vi "setPropertyIntValue.vi"(8 "error in (no error)":errorcluster, 9 "Property Value in":i32, 10 "Property Name in":string, 11 "IPropertyObject in":refnum<class "IPropertyObject.lvclass">) -> (0 "error out":errorcluster, 1 "Property Value out":i32, 2 "Property Name out":string, 3 "IPropertyObject out":refnum<class "IPropertyObject.lvclass">)   [LabVIEW 2022 SP3, in "openDAQ.lvlib" / "IBaseObject.lvlib" / "IPropertyObject.lvlib" / "IPropertyObject.lvclass"]
uses:
  <instrlib>/openDAQ/Public/Classes/IPropertyObject/IPropertyObject.lvclass
  C:/Program Files (x86)/National Instruments/LabVIEW 2022/instr.lib/openDAQ/Public/Classes/IBaseObject/IBaseObject.lvclass
  <instrlib>/openDAQ/Public/Classes/IBaseObject/IBaseObject.lvclass/IBaseObject.ctl
  <instrlib>/openDAQ/Public/Classes/IBaseObject/Accessor/Read reference.vi
  <instrlib>/openDAQ/Public/Classes/IBaseObject/Accessor/Write reference.vi
  <instrlib>/openDAQ/Public/Classes/daqCoreTypes/IInteger/IInteger.lvclass
  <instrlib>/openDAQ/Public/Classes/daqCoreTypes/IString/IString.lvclass
  <instrlib>/openDAQ/Binaries/Windows/x86/copendaq32.dll
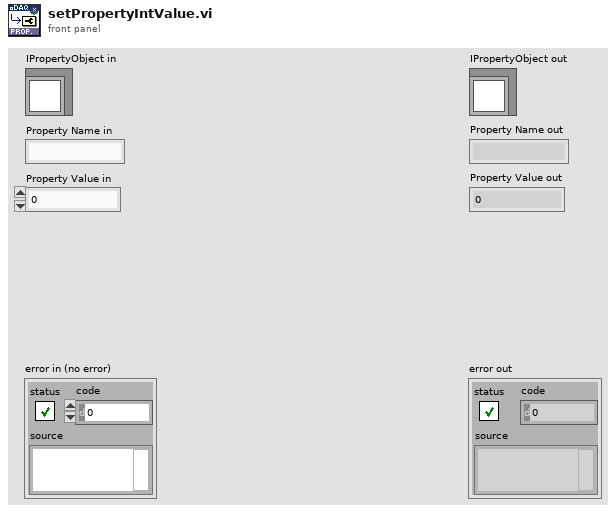
[diagram p1: front panel]
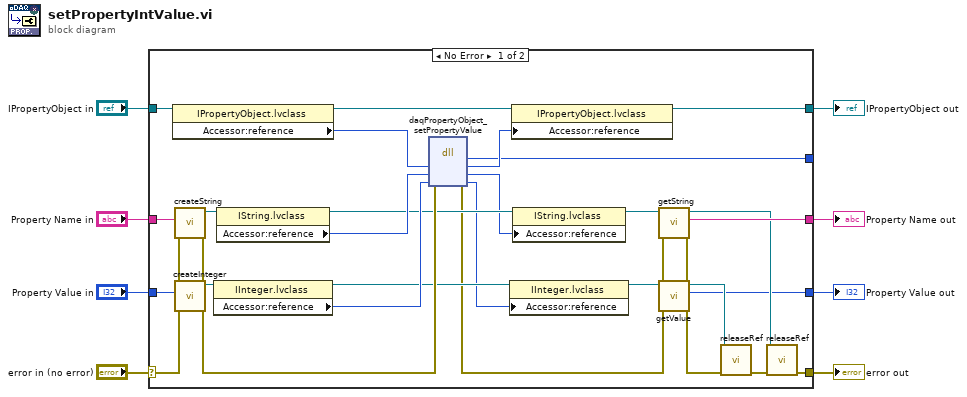
[diagram p0: block diagram]
diagram:
  n1 = case shown="No Error" "error in (no error)" {
    selector: "error in (no error)" -> [w17 w42]
    tunnel: [w25 w42] -> w7
    tunnel: [w33 w41] -> w5
    tunnel: "IPropertyObject in" -> [w36 w41]
    tunnel: "Property Name in" -> [w31 w40]
    tunnel: [w26 w40] -> w3
    tunnel: "Property Value in" -> [w18 w39]
    tunnel: [w10 w39] -> w1
    tunnel: [w9 _] -> _
    frame No Error {
      n2 = property class="IPropertyObject.lvclass"(reference=w36) -> (reference out=w34:refnum<class "IPropertyObject.lvclass">, "Accessor:reference"=w35:i64)  [unwired: 1 in, 1 out]
      n3 = call <instrlib>:"createInteger.vi"("error in (no error)"=w17, "Value"=w18) -> ("error out"=w16:errorcluster, "IInteger out"=w15:refnum<class "IInteger.lvclass">)  [unwired: 8 in]
      n4 = call <instrlib>:"createString.vi"("error in (no error)"=w16, "String"=w31) -> ("error out"=w38:errorcluster, "IString out"=w30:refnum<class "IString.lvclass">)  [unwired: 8 in]
      n5 = property class="IInteger.lvclass"(reference=w15) -> (reference out=w22:refnum<class "IInteger.lvclass">, "Accessor:reference"=w37:i64)  [unwired: 1 in, 1 out]
      n6 = property class="IString.lvclass"(reference=w30) -> (reference out=w28:refnum<class "IString.lvclass">, "Accessor:reference"=w29:i64)  [unwired: 1 in, 1 out]
      n7 = dll-call lib="C:/Program Files (x86)/National Instruments/LabVIEW 2022/instr.lib/openDAQ/Binaries/Windows/x86/copendaq*.*" fn="daqPropertyObject_setPropertyValue"(error in=w38, "config"=w35, "propertyName"=w29, "value"=w37) -> (error out=w13:errorcluster, "return type"=w9:u32, "config"=w32:i64, "propertyName"=w23:i64, "value"=w19:i64)  [unwired: 2 in, 1 out]
      n8 = property class="IInteger.lvclass"(reference=w22, "Accessor:reference"=w19) -> (reference out=w14:refnum<class "IInteger.lvclass">)  [unwired: 1 in, 1 out]
      n9 = property class="IPropertyObject.lvclass"(reference=w34, "Accessor:reference"=w32) -> (reference out=w33:refnum<class "IPropertyObject.lvclass">)  [unwired: 1 in, 1 out]
      n10 = property class="IString.lvclass"(reference=w28, "Accessor:reference"=w23) -> (reference out=w27:refnum<class "IString.lvclass">)  [unwired: 1 in, 1 out]
      n11 = call <instrlib>:"getValue.vi"("error in (no error)"=w13, "IInteger in"=w14) -> ("error out"=w12:errorcluster, "Value out"=w10:i32, "IInteger out"=w11:refnum<class "IInteger.lvclass">)  [unwired: 7 in]
      n12 = call <instrlib>:"getString.vi"("error in (no error)"=w12, "IString in"=w27) -> ("error out"=w21:errorcluster, "String out"=w26:string, "IString out"=w24:refnum<class "IString.lvclass">)  [unwired: 7 in]
      n13 = call-dynamic "releaseRef.vi"("error in (no error)"=w21, "IBaseObject in"=w11) -> ("error out"=w20:errorcluster)  [unwired: 9 in]
      n14 = call-dynamic "releaseRef.vi"("error in (no error)"=w20, "IBaseObject in"=w24) -> ("error out"=w25:errorcluster)  [unwired: 9 in]
    }
    frame Error {
    }
  }
  "error out" <- w7
  "IPropertyObject out" <- w5
  "Property Name out" <- w3
  "Property Value out" <- w1
